vi "macro_Ramsete_Execute_ENG.vi"   [LabVIEW 2019, in "Trajectory_Library.lvlib"]
uses:
  Trajectory_Library.lvlib
types:
  T1 = typedef "Trajectory_Library.lvlib/RAMSETE_EXE_TUNING.ctl" = cluster{"B":dbl, "Zeta":dbl, "X Tolerance M":dbl, "Y Tolerance M":dbl, "Heading Tolerance RAD":dbl, "Track Width M":dbl, "Max Speed M/S":dbl}
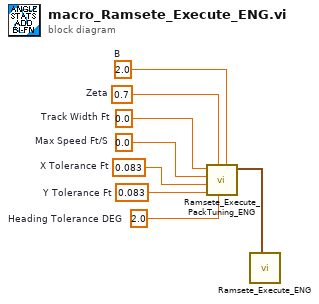
[diagram p0: block diagram]
diagram:
  w1 = 0.0  # Track Width Ft
  w2 = 0.0  # Max Speed Ft/S
  w3 = 0.083  # X Tolerance Ft
  w4 = 0.083  # Y Tolerance Ft
  w5 = 0.7  # Zeta
  w6 = 2.0  # Heading Tolerance DEG
  w7 = 2.0  # B
  n1 = call "Ramsete_Execute_PackTuning_ENG.vi"("B"=w7, "Heading Tolerance DEG"=w6, "Zeta"=w5, "Y Tolerance Ft"=w4, "X Tolerance Ft"=w3, "Max Speed Ft/S"=w2, "Track Width Ft"=w1) -> ("RAMSETE_EXE_TUNING"=w8:T1)  [unwired: 4 in]
  n2 = call "Ramsete_Execute_ENG.vi"("RAMSETE_EXE_TUNING"=w8) -> ()  [unwired: 6 in, 5 out]
